vi "Create State.vi"(8 "error in (no error)":errorcluster, 11 "Model in":refnum<class "Model.lvclass">) -> (0 "error out":errorcluster, 2 "State":refnum<class "State.lvclass">, 3 "Model out":refnum<class "Model.lvclass">)   [LabVIEW 2015, in "Model.lvclass"]
uses:
  Model.lvclass
  States/State/State.lvclass
  Model.lvclass/Model.ctl
  States/State Factory/State Factory.lvclass
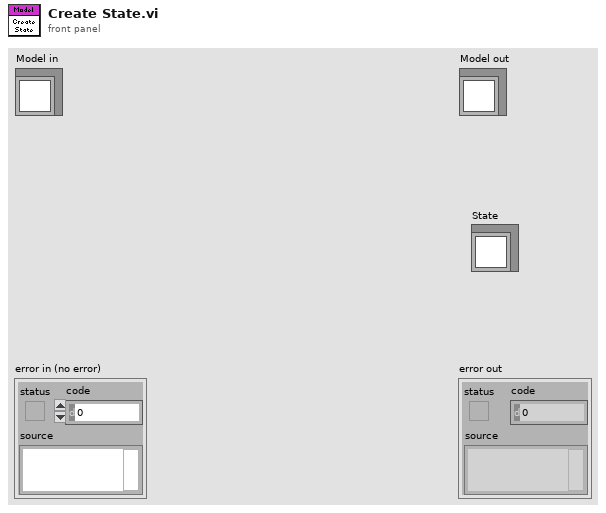
[diagram p1: front panel]
types:
  T1 = typedef "FAMT Typedefs.lvlib/State Types.ctl" = enum16{"Offline State", "Fault State", "Standby State", "Disabled State", "Enabled State", "Wait For User Input State", "Perform Open Loop Scan State", "Perform Closed Loop Scan State"}
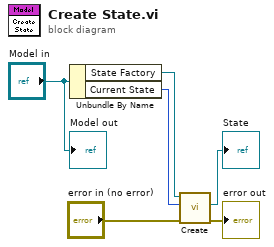
[diagram p0: block diagram]
diagram:
  n1 = Unbundle By Name("Model in") -> ("State Factory"=w5:refnum<class "State Factory.lvclass">, "Current State"=w4:T1)
  n2 = call-dynamic "Create.vi"("error in (no error)"="error in (no error)", "State Types"=w4, "State Factory in"=w5) -> ("error out"=→"error out":errorcluster, "State"=→"State":refnum<class "State.lvclass">)  [unwired: 6 in, 1 out]
  "Model out" <- "Model in"
